vi "TEMOCR-Create Stimuli.vi"(0 "AO":T2, 11 "error in (no error)":errorcluster, 12 "Step In":T1) -> (13 "finished":bool, 14 "Step":T1, 15 "error out":errorcluster)   [LabVIEW 2015]
uses:
  Typedefs/TEMOCR-AO Data.ctl
  Typedefs/TEMOCR-Sequence Step.ctl
  <vilib>/Analysis/NI_AALBase.lvlib
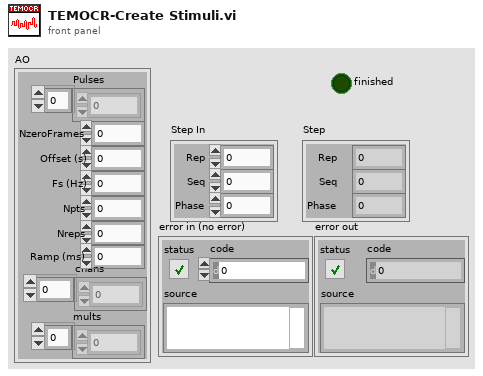
[diagram p1: front panel]
types:
  T1 = typedef "TEMOCR-Sequence Step.ctl" = cluster{"Rep":i32, "Seq":i32, "Phase":i32}
  T2 = typedef "TEMOCR-AO Data.ctl" = cluster{"Pulses":dbl[], "Fs (Hz)":dbl, "Npts":i32, "mults":dbl[], "chans":i32[], "Nreps":i32, "NzeroFrames":i32, "Offset (s)":dbl, "Ramp (ms)":dbl}
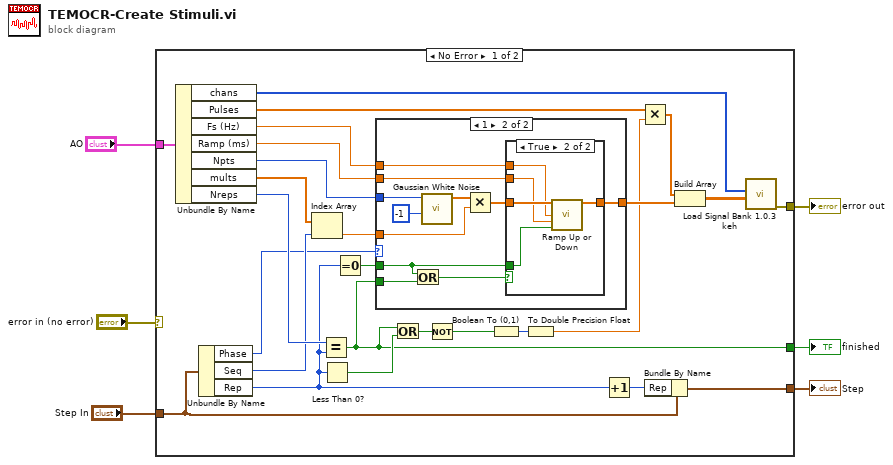
[diagram p0: block diagram]
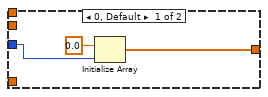
[diagram p2: hidden frame]
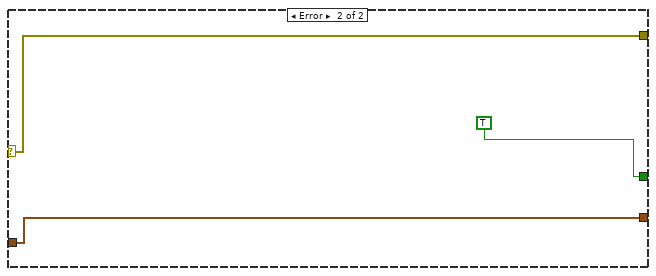
[diagram p4: hidden frame]
diagram:
  n1 = case shown="No Error" "error in (no error)" {
    selector: "error in (no error)" -> [_ w55]
    tunnel: "AO" -> [w32 _]
    tunnel: [w27 w55] -> w5
    tunnel: "Step In" -> [w24 w53]
    tunnel: [w22 w53] -> w2
    tunnel: [w9 TRUE] -> w1
    frame No Error {
      n2 = Unbundle By Name(w32) -> ("chans"=w28:i32[], "Pulses"=w18:dbl[], "Fs (Hz)"=w12:dbl, "Ramp (ms)"=w14:dbl, "Npts"=w31:i32, "mults"=w25:dbl[], "Nreps"=w26:i32)
      n3 = Unbundle By Name(w24) -> ("Phase"=w20:i32, "Seq"=w21:i32, "Rep"=w11:i32)
      n4 = Index Array(array=w25, index=w21) -> (element=w30:dbl)
      n5 = Equal?(x=w26, y=w11) -> (x = y?=w9:bool)
      n6 = Less Than 0?(x=w11) -> (x < 0?=w10:bool)
      n7 = Equal To 0?(x=w11) -> (x = 0?=w13:bool)
      n8 = case shown="1" w20 {
        tunnel: w31 -> [w35 w45]
        tunnel: w30 -> [_ w46]
        tunnel: [w33 w40] -> w29
        tunnel: w9 -> [_ w37]
        tunnel: w14 -> [_ w42]
        tunnel: w13 -> [_ w38]
        tunnel: w12 -> [_ w39]
        frame 0, Default {
          n9 = Initialize Array(0.0 ("element"), w35) -> (w33:dbl[])
        }
        frame 1 {
          n10 = Or(x=w38, y=w37) -> (x .or. y?=w36:bool)
          n11 = call <vilib>:"Gaussian White Noise.vi"("seed"=-1, "samples"=w45) -> ("Gaussian noise pattern"=w43:dbl[])  [unwired: 8 in, 1 out]
          n12 = Multiply(x=w43, y=w46) -> (x*y=w41:dbl[])
          n13 = case shown="True" w36 {
            tunnel: w42 -> [_ w48]
            tunnel: w41 -> [w47 w51]
            tunnel: [w47 w50] -> w40
            tunnel: w39 -> [_ w49]
            tunnel: w38 -> [_ w52]
            frame False {
            }
            frame True {
              n14 = call "Ramp Up or Down.vi"("Array"=w51, "Sampling rate (Hz)"=w49, "Ramp (ms)"=w48, "Ramp up?"=w52) -> ("Ramped array"=w50:dbl[])  [unwired: 10 in, 1 out]
            }
          }
        }
      }
      n15 = Or(x=w9, y=w10) -> (x .or. y?=w8:bool)
      n16 = Not(x=w8) -> (.not. x?=w7:bool)
      n17 = Boolean To (0,1)(Boolean=w7) -> (0, 1=w16:i16)
      n18 = To Double Precision Float(number=w16) -> (double precision float=w15:dbl)
      n19 = Increment(x=w11) -> (x+1=w23:i32)
      n20 = Multiply(x=w18, y=w15) -> (x*y=w17:dbl[])
      n21 = Bundle By Name(cluster=w24, "Rep"=w23) -> (w22:T1)
      n22 = Build Array(w17, w29) -> (w19:dbl[][])
      n23 = call "Load Signal Bank 1.0.3 keh.vi"("Input array"=w19, "Active AO Array"=w28) -> ("error out"=w27:errorcluster)  [unwired: 7 in, 2 out]
    }
    frame Error {
    }
  }
  "error out" <- w5
  "Step" <- w2
  "finished" <- w1
